vi "Add DID.vi"(8 "error in (no error)":errorcluster, 11 "Node Ptr":u64 format="%.0x") -> (0 "error out":errorcluster)   [LabVIEW 2013, in "Diagnostics Addon System Explorer.lvlib"]
uses:
  Diagnostics Addon System Explorer.lvlib
  <vilib>/NI Veristand/Custom Device API/Custom Device API.lvlib
  Shared/Diagnostics Addon Shared.lvlib
  <vilib>/NI Veristand/Custom Device Tools/Custom Device Utility Library/Custom Device Utility Library.lvlib
panel:
  in  "Tag":string
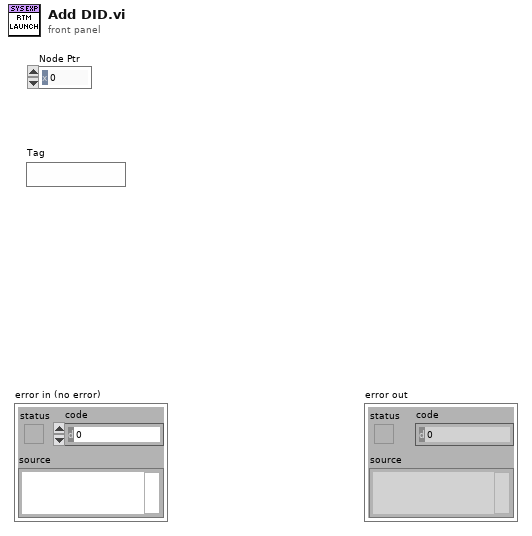
[diagram p1: front panel]
types:
  T1 = typedef "Custom Device API.lvlib/Custom Device Item Ref.ctl" = u64
  T2 = typedef "Custom Device API.lvlib/Custom Device Item Info.ctl" = cluster{"Name":string, "Is Channel":bool, "GUID":string, "Is Waveform":bool}
  T3 = typedef "Diagnostics Addon Shared.lvlib/DIDPID Parameters.ctl" = cluster{"Name":string, "Description":string, "ID":u16, "Signals":T4[]}
  T4 = typedef "Diagnostics Addon Shared.lvlib/DIDPID Signal Parameters.ctl" = cluster{"Start Bit":u8, "Length":u8, "Scaling Factor":dbl, "Scaling Offset":dbl, "Minimum":dbl, "Maximum":dbl, "Data Type":u32, "Byte Order":u32, "Default Value":dbl, "Name":string, "Units":string, "Description":string}
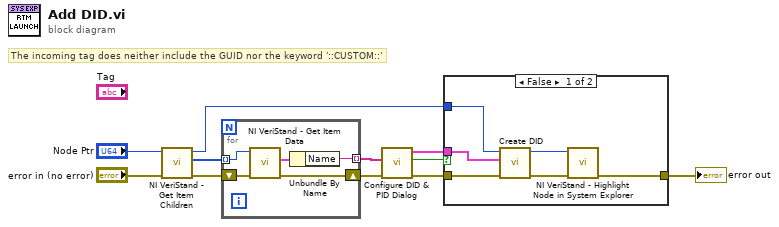
[diagram p0: block diagram]
diagram:
  # "The incoming tag does neither include the GUID nor the keyword '::CUSTOM::'"
  n1 = call <vilib>:"NI VeriStand - Get Item Children.vi"("error in (no error)"="error in (no error)", "Item Ref in"="Node Ptr") -> ("error out"=w9:errorcluster, "Child Refs"=w2:T1[], "Item Ref out"=w1:T1)  [unwired: 6 in, 1 out]
  n2 = for {
    tunnel: [w14] -> w8 mode=indexing
    shift-right: [w13] -> w7
    shift-left: w9 -> [w15]
    tunnel: w2 -> [w12] mode=indexing
    n3 = call <vilib>:"NI VeriStand - Get Item Data.vi"("error in (no error)"=w15, "Item Ref in"=w12) -> ("error out"=w13:errorcluster, "Item Info"=w16:T2)  [unwired: 8 out]
    n4 = Unbundle By Name(w16) -> ("Name"=w14:string)
  }
  n5 = call "Configure DID & PID Dialog.vi"("error in (no error)"=w7, "Existing PIDs"=w8) -> ("error out"=w5:errorcluster, "Cancel PID?"=w6:bool, "Parameters Out"=w4:T3)  [unwired: 7 in]
  n6 = case shown="False" w6 {
    tunnel: w5 -> [w22 w23]
    tunnel: w1 -> [w21 _]
    tunnel: w4 -> [w20 _]
    tunnel: [w18 w23] -> w3
    frame False {
      n7 = call "Create DID.vi"("error in (no error)"=w22, "DIDPID"=w20, "Section Ptr"=w21) -> ("error out"=w19:errorcluster, "Parent Ref out"=w17:T1)  [unwired: 7 in]
      n8 = call <vilib>:"NI VeriStand - Highlight Node in System Explorer.vi"("error in (no error)"=w19, "Item Ref in"=w17) -> ("error out"=w18:errorcluster)  [unwired: 8 in, 1 out]
    }
    frame True {
    }
  }
  "error out" <- w3
